vi "LowPassFilter.vi"(8 "input variable":dbl, 9 "Tf[s]":dbl, 10 "Ts[s]":dbl, 11 "u_k":dbl) -> (3 "output variable":dbl)   [LabVIEW 2019]
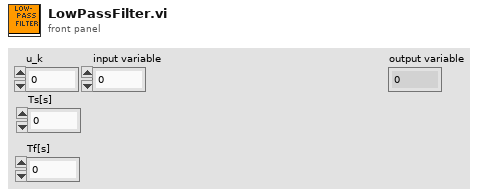
[diagram p1: front panel]
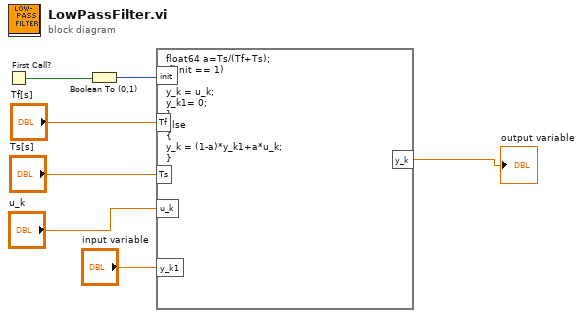
[diagram p0: block diagram]
diagram:
  n1 = First Call?() -> (First Call?: T/F=w7:bool)
  n2 = Boolean To (0,1)(Boolean=w7) -> (0, 1=w3:i16)
  n3 = formula code="float64 a=Ts/(Tf+Ts);\nif(init == 1)\n{\ny_k = u_k;\ny_k1= 0;\n}\nelse\n{\ny_k = (1-a)*y_k1+a*u_k;\n}"("init"=w3, "Tf"="Tf[s]", "Ts"="Ts[s]", "u_k"="u_k", "y_k1"="input variable") -> ("y_k"=→"output variable":dbl)
